vi "Img Overlay Bitmap.vi"(8 "error in (no error)":errorcluster, 9 "Size":cluster{"X Resolution":i32, "Y Resolution":i32}, 10 "Bitmap":u32[][](array[colorbox]), 11 "Image":T1) -> (0 "error out":errorcluster, 3 "Image Dst Out":T1)   [LabVIEW 2018, in "Image Process.lvclass"]
uses:
  Image Process.lvclass
  <vilib>/vision/Image Controls.llb/IMAQ Image.ctl
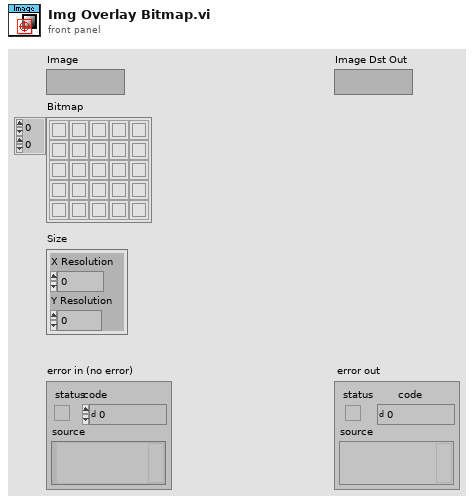
[diagram p1: front panel]
types:
  T1 = typedef "IMAQ Image.ctl" = refnum<image>
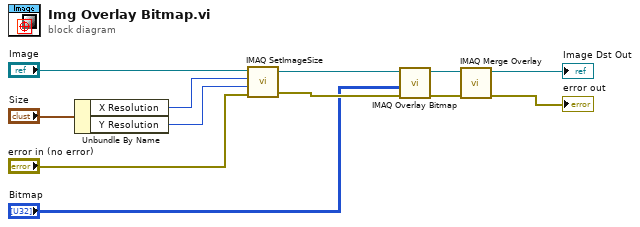
[diagram p0: block diagram]
diagram:
  n1 = Unbundle By Name("Size") -> ("X Resolution"=w4:i32, "Y Resolution"=w3:i32)
  n2 = call "IMAQ SetImageSize"("error in (no error)"="error in (no error)", "Y Resolution"=w3, "X Resolution"=w4, "Image"="Image") -> ("error out"=w12:errorcluster, "Image Out"=w11:T1)  [unwired: 1 in]
  n3 = call "IMAQ Overlay Bitmap"("error in (no error)"=w12, "Bitmap"="Bitmap", "Image"=w11) -> ("error out"=w9:errorcluster, "Image Out"=w10:T1)  [unwired: 7 in]
  n4 = call "IMAQ Merge Overlay"("error in (no error)"=w9, "Image Src"=w10) -> ("error out"=→"error out":errorcluster, "Image Dst Out"=→"Image Dst Out":T1)  [unwired: 8 in]
